vi "M0 Hybrid car.vi"(11 "NXT/EV3":T1) -> (3 "EV3 out":T1)   [LabVIEW 2016]
uses:
  <vilib>/NXT/Subs/LVHSConnector.ctl
  <vilib>/NXT/LegoClasses/BrickReference/BrickReference.lvclass
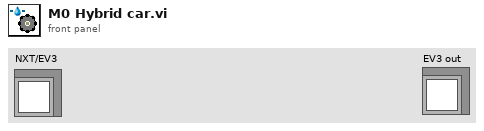
[diagram p1: front panel]
types:
  T1 = typedef "LVHSConnector.ctl" = refnum<class "BrickReference.lvclass">
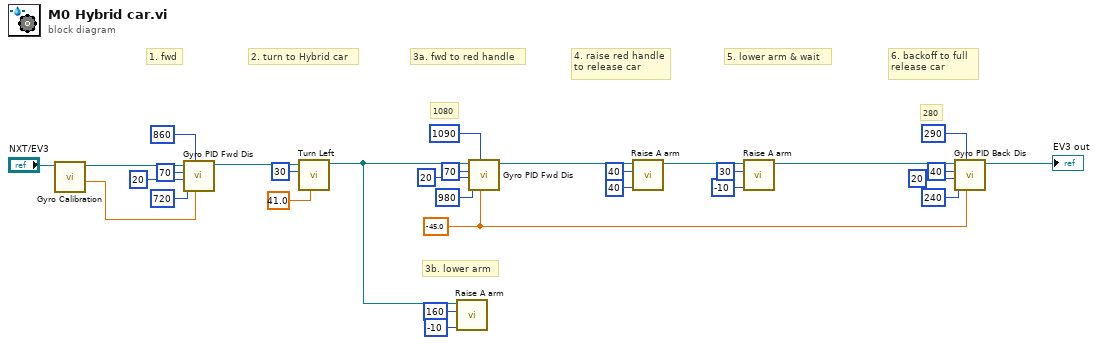
[diagram p0: block diagram]
diagram:
  w4 = sgl -45.0 ("Target angle")
  # "280"
  # "1080"
  # "6. backoff to full\nrelease car"
  # "5. lower arm & wait"
  # "4. raise red handle\nto release car"
  # "3b. lower arm"
  # "3a. fwd to red handle"
  # "2. turn to Hybrid car"
  # "1. fwd"
  n1 = call "Gyro Calibration.vi"("NXT/EV3"="NXT/EV3") -> ("Degrees"=w25:sgl, "NXT/EV3"=w30:T1)  [unwired: 6 in, 1 out]
  n2 = call "Gyro PID Fwd Dis.vi"("Target angle"=w25, "Threshold to stop"=860, "Threshold to slow"=720, "Min. speed"=20, "Max. speed"=70, "EV3 in"=w30) -> ("EV3 out"=w18:T1)  [unwired: 5 in]
  n3 = call "Turn Left.vi"("Turning angle"=sgl 41.0, "Motor B (right)"=i8 30, "EV3 in"=w18) -> ("EV3 out"=w17:T1)  [unwired: 8 in]
  n4 = call "Raise A arm.vi"("Power"=i8 -10, "Rotation"=160, "EV3 in"=w17) -> ()  [unwired: 8 in, 1 out]
  n5 = call "Gyro PID Fwd Dis.vi"("Target angle"=w4, "Threshold to stop"=1090, "Threshold to slow"=980, "Min. speed"=20, "Max. speed"=70, "EV3 in"=w17) -> ("EV3 out"=w13:T1)  [unwired: 5 in]
  n6 = call "Raise A arm.vi"("Power"=i8 40, "Rotation"=40, "EV3 in"=w13) -> ("EV3 out"=w9:T1)  [unwired: 8 in]
  n7 = call "Raise A arm.vi"("Power"=i8 -10, "Rotation"=30, "EV3 in"=w9) -> ("EV3 out"=w1:T1)  [unwired: 8 in]
  n8 = call "Gyro PID Back Dis.vi"("Target angle"=w4, "Threshold to stop"=290, "Threshold to slow"=240, "Min. speed"=20, "Max. speed"=40, "EV3 in"=w1) -> ("EV3 out"=→"EV3 out":T1)  [unwired: 5 in]
